vi "Move_Elevator.vi"(8 "error in (no error)":errorcluster, 11 "Elevator in":T1) -> (0 "error out":errorcluster, 3 "Elevator out":T1={"Door"=enum."Closed", "Person"=enum."Occupied", "Floors"={"0"=FALSE, "1"=FALSE, "2"=FALSE, "3"=FALSE}, "Up/Down/Idle"=enum."Idle", "Car Calls for Each Floor"=[FALSE, FALSE, FALSE, FALSE], "Up/Down Hall Calls for Each Floor"=[[{FALSE}, {FALSE}], [{FALSE}, {FALSE}], [{FALSE}, {FALSE}], [{FALSE}, {FALSE}], [{FALSE}, {FALSE}]]})   [LabVIEW 2026]
uses:
  Controls/Elevator_Status.ctl
  Controls/Door_Status_Enum.ctl
  Controls/Occupy_Status.ctl
  Controls/Floor_Status.ctl
  Controls/Motion_Status_Enum.ctl
  Controls/Car_Calls_Status.ctl
  Controls/Hall_Calls_Status.ctl
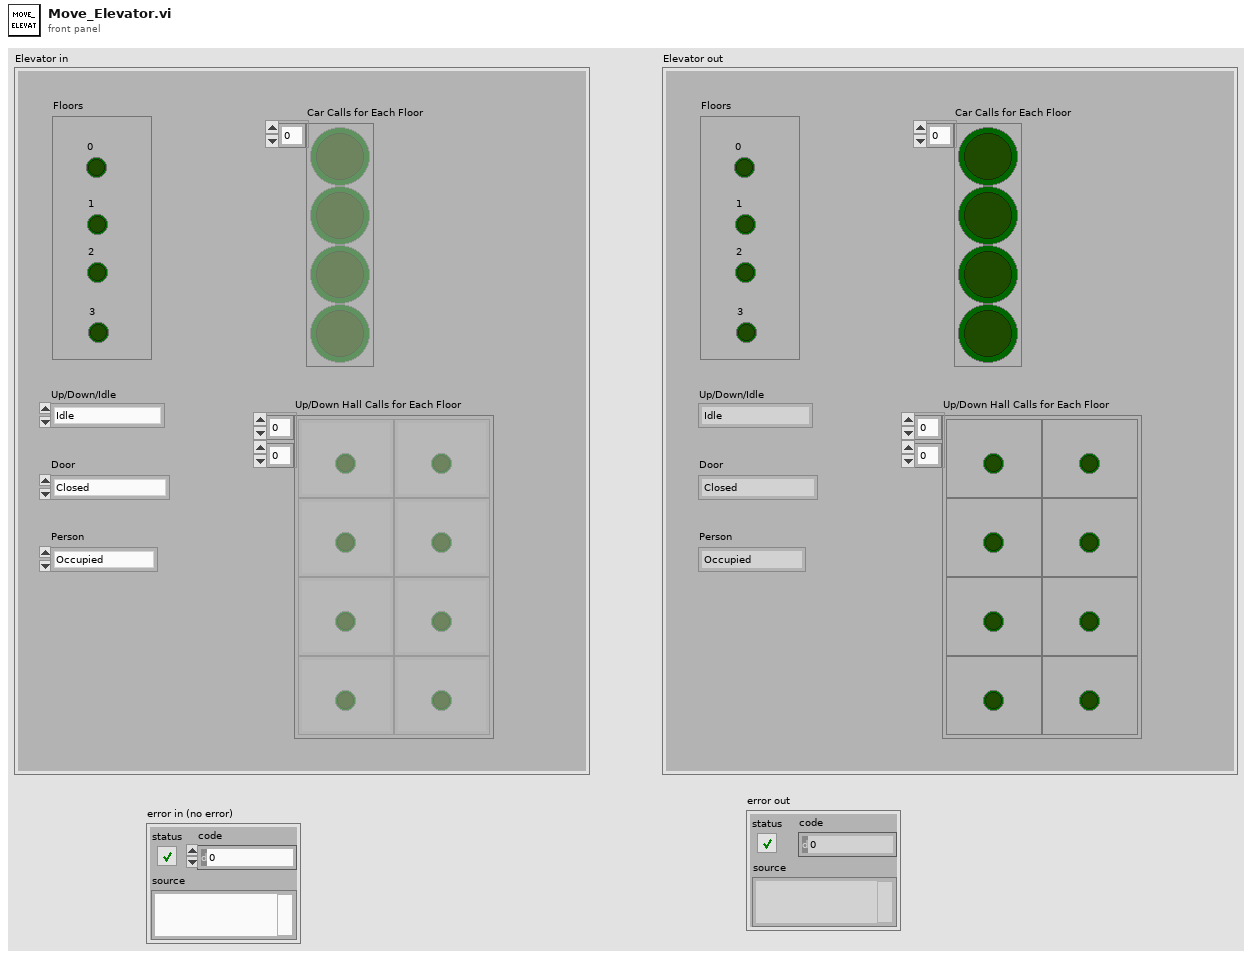
[diagram p1: front panel]
types:
  T1 = typedef "Elevator_Status.ctl" = cluster{"Door":T2, "Person":T3, "Floors":T4, "Up/Down/Idle":T5, "Car Calls for Each Floor":T6, "Up/Down Hall Calls for Each Floor":T7}
  T2 = typedef "Door_Status_Enum.ctl" = enum16{"Closed", "Open", "Opening", "Closing"}
  T3 = typedef "Occupy_Status.ctl" = enum16{"Occupied", "Empty"}
  T4 = typedef "Floor_Status.ctl" = cluster{"0":bool, "1":bool, "2":bool, "3":bool}
  T5 = typedef "Motion_Status_Enum.ctl" = enum16{"Idle", "Up", "Down"}
  T6 = typedef "Car_Calls_Status.ctl" = bool[]
  T7 = typedef "Hall_Calls_Status.ctl" = cluster{bool}[][]
  T8 = cluster{"Floors[0]":bool, "Floors[1]":bool, "Floors[2]":bool, "Floors[3]":bool}
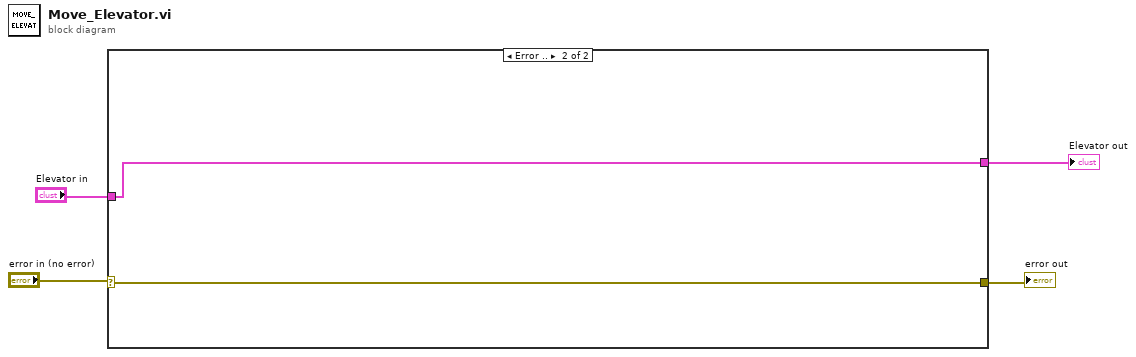
[diagram p0: block diagram]
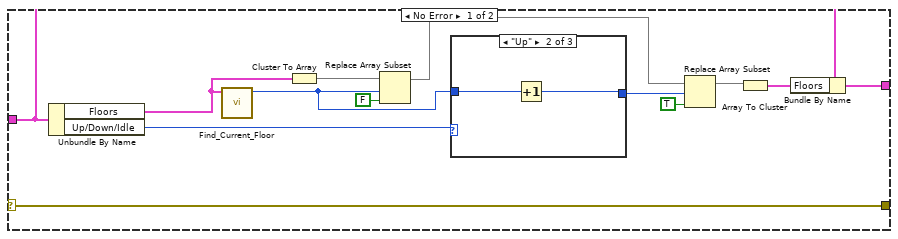
[diagram p2: hidden frame]
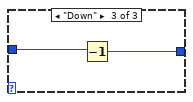
[diagram p4: hidden frame]
diagram:
  n1 = case shown="Error .." "error in (no error)" {
    selector: "error in (no error)" -> [w5 w24]
    tunnel: "Elevator in" -> [w8 w23]
    tunnel: [w6 w23] -> w3
    tunnel: [w5 w24] -> w1
    frame No Error {
      n2 = Unbundle By Name(w8) -> ("Floors"=w10:T4, "Up/Down/Idle"=w17:T5)
      n3 = call "Find_Current_Floor.vi"("Floors"=w10) -> ("Current Floor"=w13:i32)  [unwired: 9 in, 1 out]
      n4 = Cluster To Array(cluster=w10) -> (array=w14:bool[])
      n5 = Replace Array Subset(array=w14, new element=FALSE ("new element/subarray"), index=w13) -> (w12:bool[])
      n6 = case shown="\"Up\"" w17 {
        tunnel: w13 -> [w18 w20 w22]
        tunnel: [w18 w19 w21] -> w11
        frame "Idle", Default {
        }
        frame "Up" {
          n7 = Increment(x=w20) -> (x+1=w19:i32)
        }
        frame "Down" {
          n8 = Decrement(x=w22) -> (x-1=w21:i32)
        }
      }
      n9 = Replace Array Subset(array=w12, new element=TRUE ("new element/subarray"), index=w11) -> (w9:bool[])
      n10 = Array To Cluster(array=w9) -> (cluster=w7:T8)
      n11 = Bundle By Name(cluster=w8, "Floors"=w7) -> (w6:T1)
    }
    frame Error {
    }
  }
  "Elevator out" <- w3
  "error out" <- w1
